vi "TimerStimulus.vi"(6 "Enum":enum16{"Punishment", "ITI", "Response"}(ring), 8 "error in (no error)":errorcluster, 10 "Method":T1(ring)=enum."Get Elapsed Time", 11 "Stimulus in":refnum<class "Stimulus.lvclass">) -> (0 "error out":errorcluster, 1 "Timeout":bool, 2 "Time":dbl, 3 "Stimulus out":refnum<class "Stimulus.lvclass">)   [LabVIEW 2014, in "Stimulus.lvclass"]
uses:
  Stimulus.lvclass
  Stimulus.lvclass/Stimulus.ctl
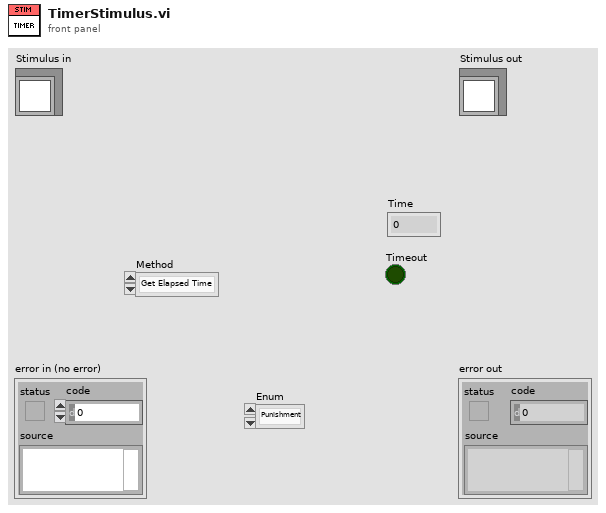
[diagram p1: front panel]
types:
  T1 = enum16{"Get Time", "Get Elapsed Time", "Reset Elapsed Time"}
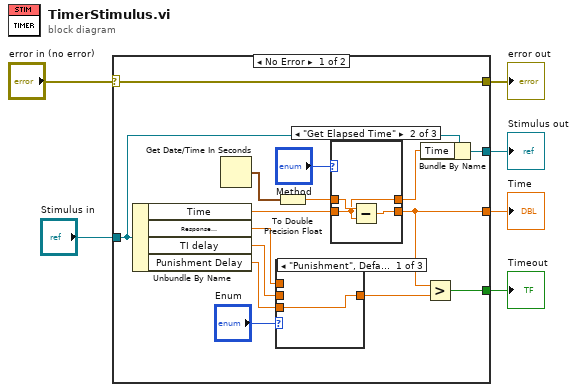
[diagram p0: block diagram]
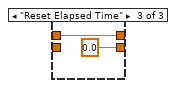
[diagram p5: hidden frame]
diagram:
  n1 = case shown="No Error" "error in (no error)" {
    selector: "error in (no error)" -> [w21 w33]
    tunnel: [w21 w33] -> w5
    tunnel: [w7 w32] -> w3
    tunnel: "Stimulus in" -> [w8 w32]
    tunnel: [w16 _] -> w2
    tunnel: [w19 _] -> w1
    frame No Error {
      n2 = Unbundle By Name(w8) -> ("Time"=w15:dbl, "Response \nperiod"=w9:dbl, "TI delay"=w12:dbl, "Punishment Delay"=w10:dbl)
      n3 = Get Date/Time In Seconds() -> (seconds since 1Jan1904=w18:timestamp)
      n4 = case shown="\"Punishment\", Default" "Enum" {
        tunnel: w12 -> [_ _ w24]
        tunnel: [w22 w23 w24] -> w11
        tunnel: w10 -> [w22 _ _]
        tunnel: w9 -> [_ w23 _]
        frame "Punishment", Default {
        }
        frame "Response" {
        }
        frame "ITI" {
        }
      }
      n5 = To Double Precision Float(number=w18) -> (double precision float=w17:dbl)
      n6 = case shown="\"Get Elapsed Time\"" "Method" {
        tunnel: w17 -> [w26 w29 w31]
        tunnel: [w26 w28 0.0] -> w16
        tunnel: w15 -> [w25 w27 _]
        tunnel: [w25 w27 w31] -> w14
        frame "Get Time", Default {
        }
        frame "Get Elapsed Time" {
          n7 = Subtract(x=w29, y=w27) -> (x-y=w28:dbl)
        }
        frame "Reset Elapsed Time" {
        }
      }
      n8 = Bundle By Name(cluster=w8, "Time"=w14) -> (w7:refnum<class "Stimulus.lvclass">)
      n9 = Greater?(x=w16, y=w11) -> (0:w19:bool)
    }
    frame Error {
    }
  }
  "error out" <- w5
  "Stimulus out" <- w3
  "Time" <- w2
  "Timeout" <- w1
